vi "Displaying a Variant in a Tree Control.vi"() -> ()   [LabVIEW 2017]
uses:
  <vilib>/National Instruments/Variant Tree Tools/Variant Tree API.lvlib
panel:
  in  "Variant":cluster{"String":string, "Array":bool[]}
  in  "Tree":string(tree)
  # "Modify this cluster, then run the application"
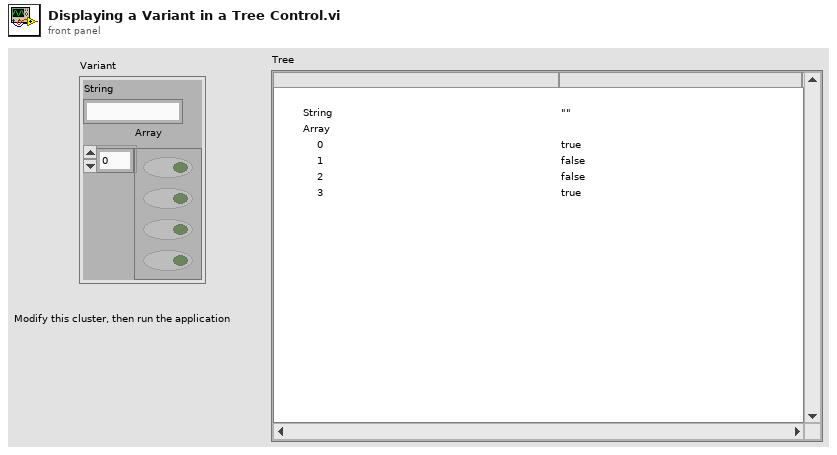
[diagram p1: front panel]
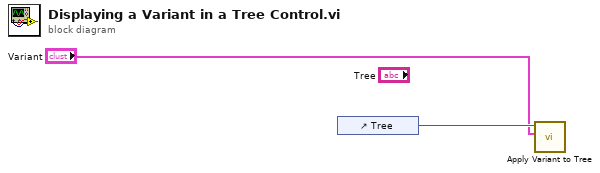
[diagram p0: block diagram]
diagram:
  n1 = control-ref of="Tree"() -> (w2:refnum<vi>)
  n2 = call <vilib>:"Apply Variant to Tree.vi"("Variant"="Variant", "TreeControl in"=w2) -> ()  [unwired: 8 in, 2 out]
